vi "special MCL.vi"() -> ()   [LabVIEW 2015]
uses:
  <vilib>/Utility/miscctls.llb/LVRowAndColumnTypeDef.ctl
panel:
  in  "path to PNG file":path=path "C:/ProjectLocker/NHMFL/LANL/Libraries/Mag Lab Measure/Queued Listbox/Parameters.png"
  out "2D Picture":picture
  in  "Preferences Button":bool
  in  "Numeric":i32
  in  "Indent":i32=5
  in  "new element/subarray":i32
  in  "Active Cell:Active Cell":T1
  out "Item Symbols":i32[](array[numeric])
  out "Array - Numeric":i32[](array[numeric])
  in  "tree listbox":i32[](listbox) caption="Double-click an example to open it."
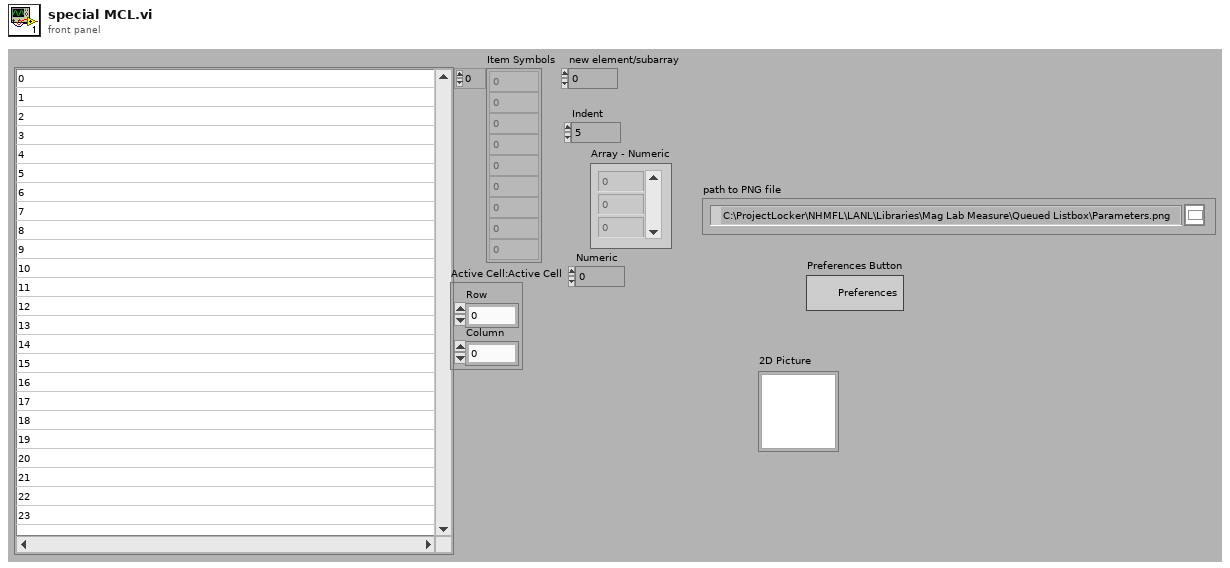
[diagram p1: front panel]
types:
  T1 = typedef "LVRowAndColumnTypeDef.ctl" = cluster{"Row":i32, "Column":i32}
  T2 = typedef "imagedata.ctl" = cluster{"image type":i32, "image depth":i32, "image":u8[], "mask":u8[], "colors":u32[], "Rectangle":cluster{"left":i16, "top":i16, "right":i16, "bottom":i16}}
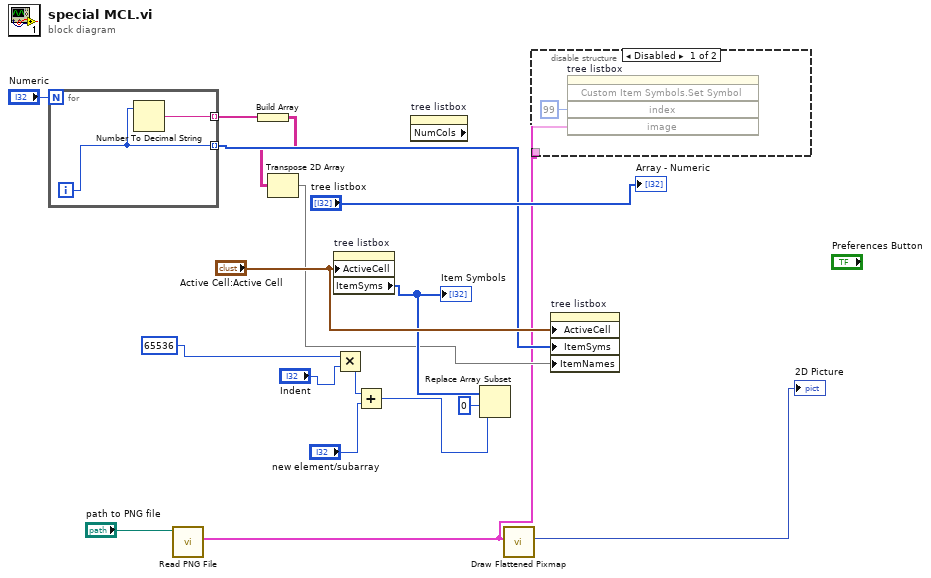
[diagram p0: block diagram]
diagram:
  n1 = for {
    N: "Numeric" -> [_]
    tunnel: [w19] -> w7 mode=indexing
    tunnel: [w18] -> w6 mode=indexing
    i -> [w19]
    n2 = Number To Decimal String(number=w19) -> (decimal integer string=w18:string)  [unwired: 1 in]
  }
  n3 = call <vilib>:"Read PNG File.vi"("path to PNG file"="path to PNG file") -> ("image data"=w1:T2)  [unwired: 8 in, 2 out]
  n4 = Build Array(w6) -> (w5:string[][])
  n5 = Transpose 2D Array(2D array=w5) -> (transposed array=w4:string[][])
  n6 = property on="tree listbox" class="MCListbox (strict)"("ActiveCell"="Active Cell:Active Cell") -> ("ItemSyms"=w15:i32[])  [unwired: 2 in, 2 out]
  "Item Symbols" <- w15
  n7 = Multiply(x=65536 ("Indent"), y="Indent") -> (x*y=w9:i32)
  n8 = Add(x=w9, y="new element/subarray") -> (x+y=w12:i32)
  n9 = property on="tree listbox" class="MCListbox (strict)" props=["NumCols"]() -> ()  [unwired: 2 in, 3 out]
  n10 = Replace Array Subset(array=w15, new element=w12, index=0) -> ()  [unwired: 1 out]
  n11 = call <vilib>:"Draw Flattened Pixmap.vi"("image data"=w1) -> ("new picture"=→"2D Picture":picture)  [unwired: 8 in]
  n12 = disable-structure shown="Disabled" {
    disable-tunnel: w1 -> [w20 _]
    frame Disabled {
      n13 = invoke on="tree listbox" class="MCListbox (strict)" method="Custom Item Symbols.Set Symbol"("index"=99 ("Index"), "image"=w20) -> ()  [unwired: 3 in, 5 out]
    }
    frame Enabled {
    }
  }
  n14 = property on="tree listbox" class="MCListbox (strict)"("ActiveCell"="Active Cell:Active Cell", "ItemSyms"=w7, "ItemNames"=w4) -> ()  [unwired: 2 in, 2 out]
  "Array - Numeric" <- "tree listbox"
